vi "Measurement UI.vi"() -> ()   [LabVIEW 2021, in "Dialog Box UI.lvlib"]
uses:
  Dialog Box UI.lvlib
panel:
  in  "Clear":bool
  out "No?":bool
  out "Yes?":bool
  out "Ok?":bool
  in  "One Button DB":bool
  in  "Two Button DB":bool
  out "Selection":string
  in  "Three Button DB":bool
  out "Gender":string
  out "Location":u32(ring) items=["None", "Austin, TX", "New York City, NY", "Chicago, IL"]
  out "Name":string
  in  "Custom DB":bool
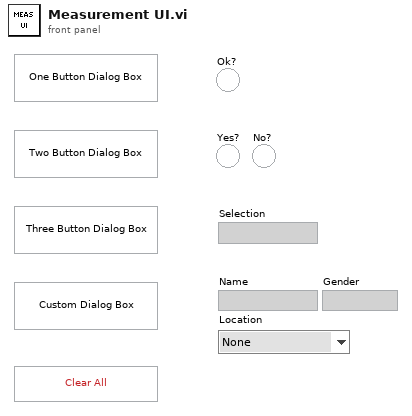
[diagram p1: front panel]
types:
  T1 = enum16{"Left Button", "Center Button", "Right Button", "Window Close"}
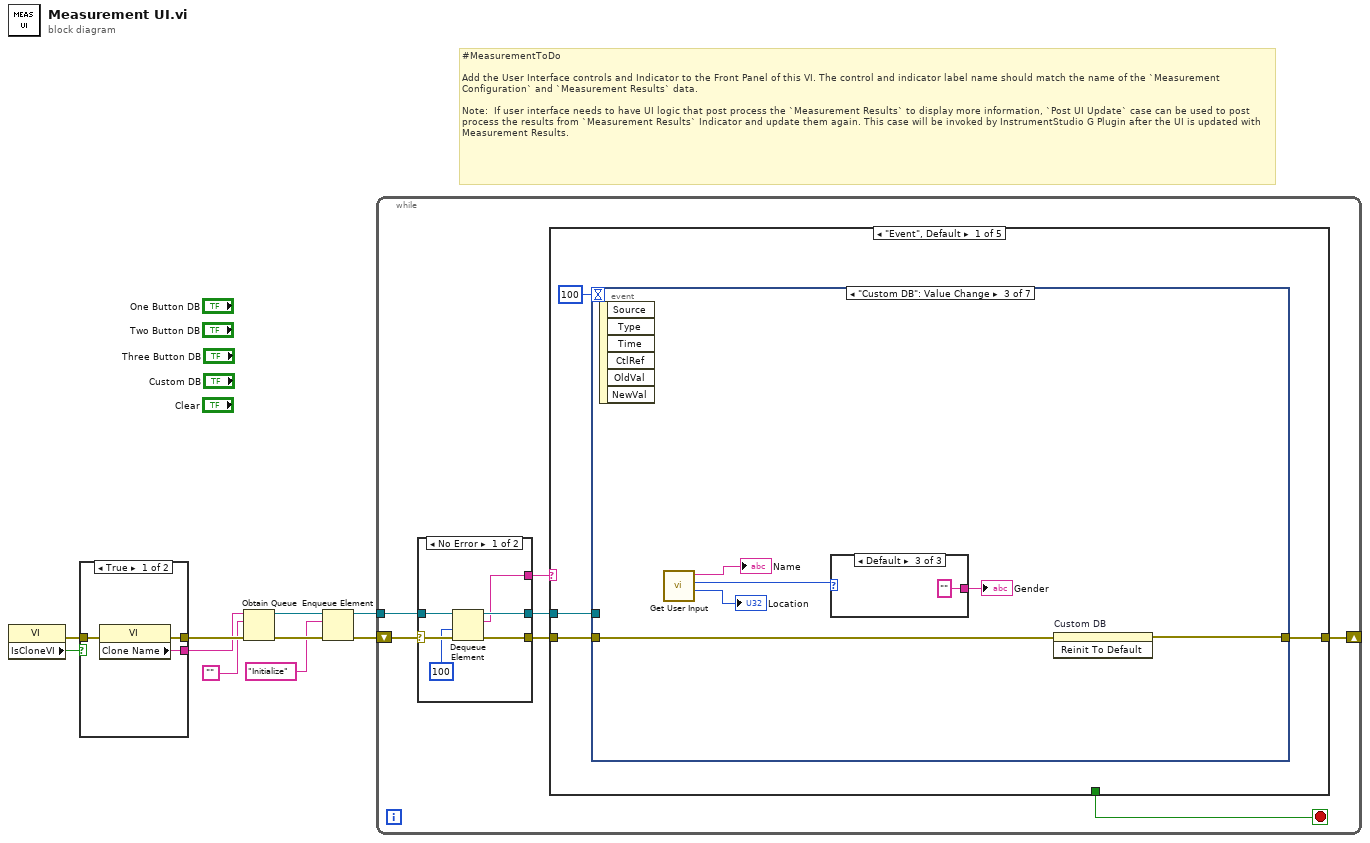
[diagram p0: block diagram]
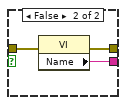
[diagram p2: hidden frame]
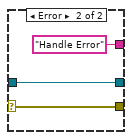
[diagram p3: hidden frame]
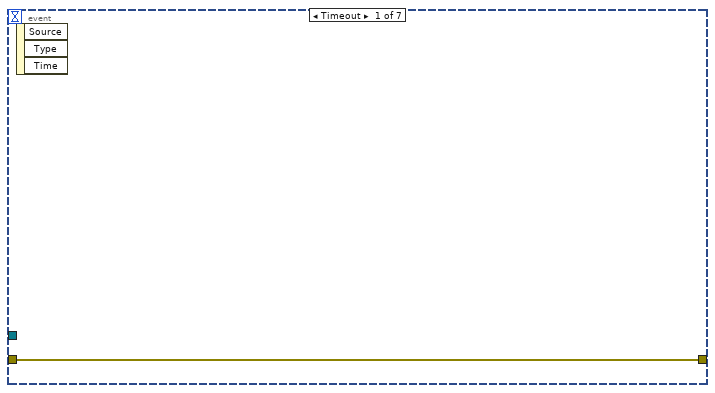
[diagram p4: hidden frame]
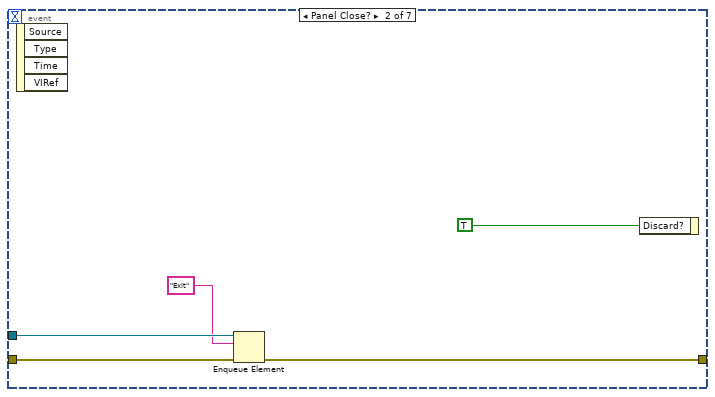
[diagram p5: hidden frame]
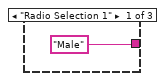
[diagram p6: hidden frame]
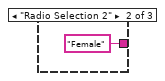
[diagram p7: hidden frame]
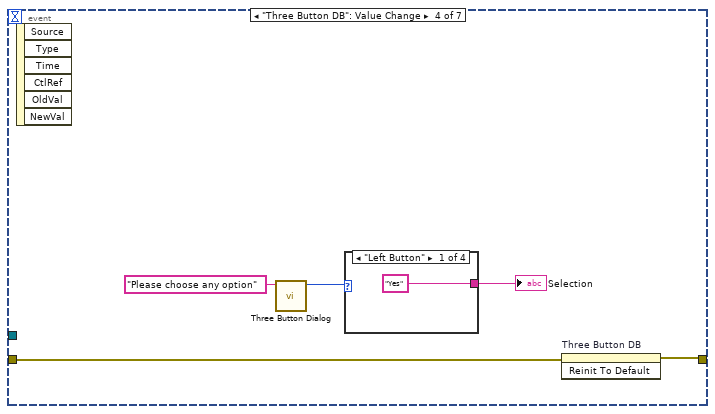
[diagram p8: hidden frame]
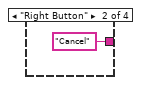
[diagram p9: hidden frame]
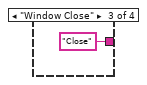
[diagram p10: hidden frame]
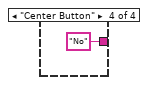
[diagram p11: hidden frame]
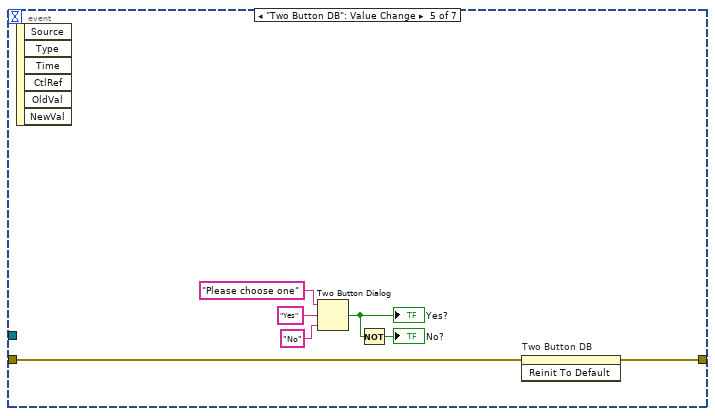
[diagram p12: hidden frame]
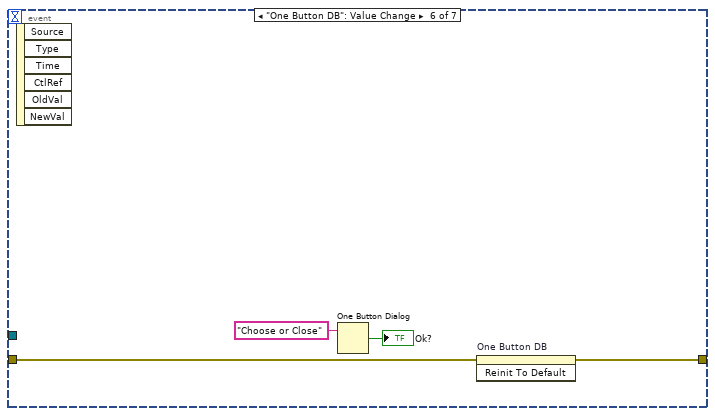
[diagram p13: hidden frame]
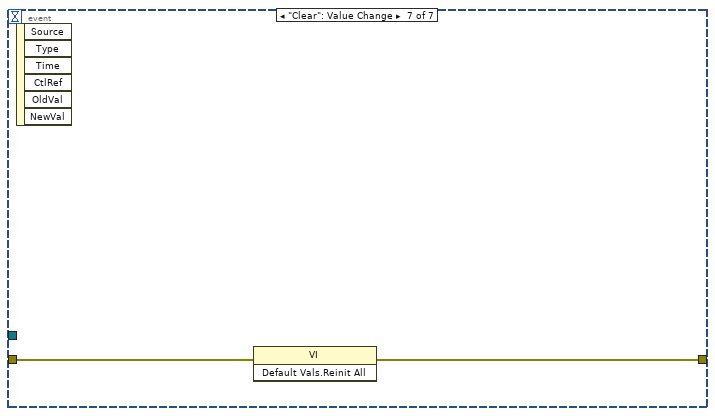
[diagram p14: hidden frame]
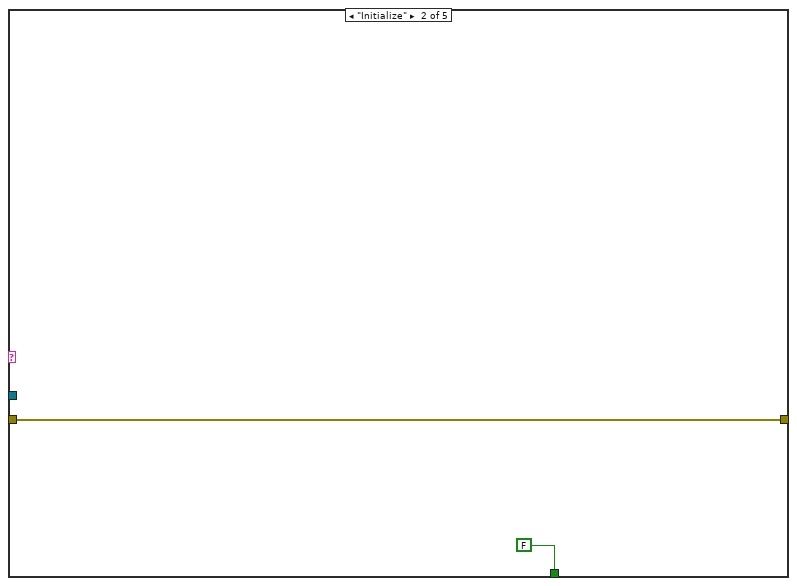
[diagram p15: hidden frame]
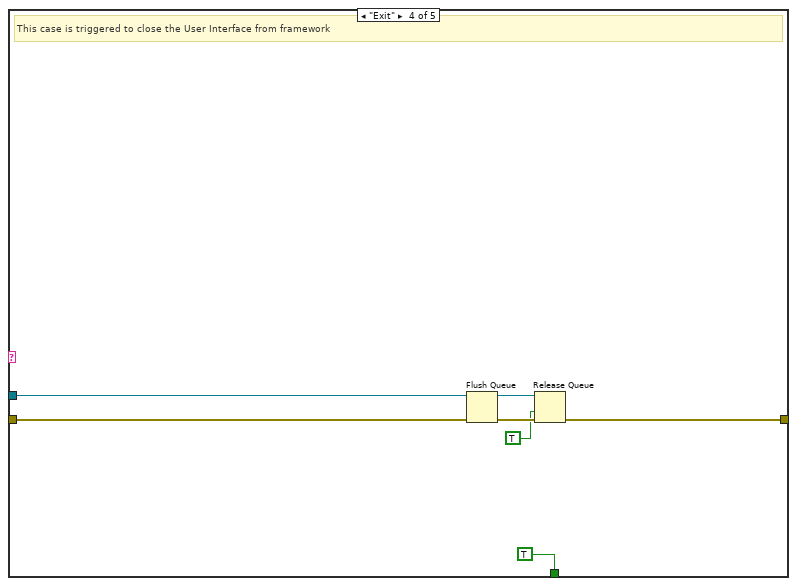
[diagram p17: hidden frame]
diagram:
  # "#MeasurementToDo  \n\nAdd the User Interface controls and Indicator to the Front Panel of this VI. The control and indicator label name should match the name of the `Measurement Configuration` and `Measurement Results` data.\n\nNote:  If user interface needs to have UI logic that post process the `Measurement Results` to display more information, `Post UI Update` case can be used to post process the results from `Measurement Results` Indicator and update them again. This case will be invoked by InstrumentStudio G Plugin after the UI is updated with Measurement Results."
  n1 = property class="VI"() -> (error out=w1:errorcluster, "IsCloneVI"=w2:bool)  [unwired: 2 in, 1 out]
  n2 = case shown="True" w2 {
    tunnel: [w13 w16] -> w10
    tunnel: [w12 w15] -> w9
    tunnel: w1 -> [w11 w14]
    frame True {
      n3 = property class="VI"(error in=w11) -> (error out=w13:errorcluster, "Clone Name"=w12:string)  [unwired: 1 in, 1 out]
    }
    frame False {
      n4 = property class="VI"(error in=w14) -> (error out=w16:errorcluster, "Name"=w15:string)  [unwired: 1 in, 1 out]
    }
  }
  n5 = Obtain Queue(name (unnamed)=w9, element data type="", error in (no error)=w10) -> (queue out=w6:refnum<queue>, error out=w8:errorcluster)  [unwired: 2 in, 1 out]
  n6 = Enqueue Element(queue=w6, element="Initialize", error in (no error)=w8) -> (queue out=w5:refnum<queue>, error out=w7:errorcluster)  [unwired: 1 in, 1 out]
  n7 = while {
    shift-right: [w18] -> _
    shift-left: w7 -> [w23]
    tunnel: w5 -> [w21]
    stop <- w17 stop-if-true
    n8 = case shown="No Error" w23 {
      selector: w23 -> [w29 w32]
      tunnel: [w28 w32] -> w22
      tunnel: w21 -> [w27 w31]
      tunnel: [w26 w31] -> w20
      tunnel: [w25 "Handle Error"] -> w19
      frame No Error {
        n9 = Dequeue Element(queue=w27, timeout in ms (-1)=100, error in (no error)=w29) -> (queue out=w26:refnum<queue>, element=w25:string, error out=w28:errorcluster)  [unwired: 1 out]
      }
      frame Error {
      }
    }
    n10 = case shown="\"Event\", Default" w19 {
      tunnel: w22 -> [w35 w75 w76 w83 w84]
      tunnel: w20 -> [w33 _ _ w81 _]
      tunnel: [w36 w75 w76 w78 w84] -> w18
      tunnel: [_ FALSE _ TRUE _] -> w17
      frame "Event", Default {
        n11 = event shown="[2] \"Custom DB\": Value Change" {
          selector: _ -> [_ _ _ _ _ _ _]
          dyn-events: _ -> [_ _ _ _ _ _ _]
          timeout: 100 -> [_ _ _ _ _ _ _]
          tunnel: [w37 w40 w47 w53 w65 w69 w72] -> w36
          tunnel: w35 -> [w37 w41 w48 w52 w66 w70 w73]
          tunnel: w33 -> [_ w39 _ _ _ _ _]
          event Timeout {
            n12 = event-data() -> ()  [unwired: 1 in, 3 out]
          }
          event Panel Close? {
            n13 = event-data() -> ()  [unwired: 1 in, 4 out]
            n14 = Enqueue Element(queue=w39, element="Exit", error in (no error)=w41) -> (error out=w40:errorcluster)  [unwired: 1 in, 2 out]
            n15 = event-data("Discard?"=TRUE) -> ()  [unwired: 1 in, 1 out]
          }
          event "Custom DB": Value Change {
            n16 = event-data() -> ()  [unwired: 1 in, 6 out]
            n17 = call "Get User Input.vi"() -> ("Location"=→"Location":u32, "Gender"=w44:enum32{"Radio Selection 1", "Radio Selection 2"}, "Name"=→"Name":string)  [unwired: 9 in]
            n18 = case shown="Default" w44 {
              tunnel: ["Male" ("Gender") "Female" ("Gender") "" ("Gender")] -> w43
              frame "Radio Selection 1" {
              }
              frame "Radio Selection 2" {
              }
              frame Default {
              }
            }
            "Gender" <- w43
            n19 = invoke on="Custom DB" class="Bool" method="Reinit To Default"(error in=w48) -> (error out=w47:errorcluster)  [unwired: 2 in, 2 out]
          }
          event "Three Button DB": Value Change {
            n20 = event-data() -> ()  [unwired: 1 in, 6 out]
            n21 = call <vilib>:"Three Button Dialog.vi"("message"="Please choose any option") -> ("Which Button?"=w55:T1)  [unwired: 10 in]
            n22 = case shown="\"Left Button\"" w55 {
              tunnel: ["Yes" ("Selection") "Cancel" ("Selection") "Close" ("Selection") "No" ("Selection")] -> w54
              frame "Left Button" {
              }
              frame "Right Button" {
              }
              frame "Window Close" {
              }
              frame "Center Button" {
              }
            }
            "Selection" <- w54
            n23 = invoke on="Three Button DB" class="Bool" method="Reinit To Default"(error in=w52) -> (error out=w53:errorcluster)  [unwired: 2 in, 2 out]
          }
          event "Two Button DB": Value Change {
            n24 = event-data() -> ()  [unwired: 1 in, 6 out]
            n25 = Two Button Dialog(message="Please choose one", 1:"No" ("F button name (\"Cancel\")"), 2:"Yes" ("T button name (\"OK\")")) -> (T button?=w62:bool)
            "Yes?" <- w62
            n26 = Not(x=w62) -> (.not. x?=→"No?":bool)
            n27 = invoke on="Two Button DB" class="Bool" method="Reinit To Default"(error in=w66) -> (error out=w65:errorcluster)  [unwired: 2 in, 2 out]
          }
          event "One Button DB": Value Change {
            n28 = event-data() -> ()  [unwired: 1 in, 6 out]
            n29 = One Button Dialog(message="Choose or Close") -> (true=→"Ok?":bool)  [unwired: 1 in]
            n30 = invoke on="One Button DB" class="Bool" method="Reinit To Default"(error in=w70) -> (error out=w69:errorcluster)  [unwired: 2 in, 2 out]
          }
          event "Clear": Value Change {
            n31 = event-data() -> ()  [unwired: 1 in, 6 out]
            n32 = invoke class="VI" method="Default Vals.Reinit All"(error in=w73) -> (error out=w72:errorcluster)  [unwired: 2 in, 2 out]
          }
        }
      }
      frame "Initialize" {
      }
      frame "Post UI Update" {
        # "This case will be triggered, after framework updates the User interface with result values."
      }
      frame "Exit" {
        # "This case is triggered to close the User Interface from framework"
        n33 = Flush Queue(queue=w81, error in (no error)=w83) -> (queue out=w80:refnum<queue>, error out=w79:errorcluster)  [unwired: 1 out]
        n34 = Release Queue(queue=w80, force destroy? (F)=TRUE, error in (no error)=w79) -> (error out=w78:errorcluster)  [unwired: 2 out]
      }
      frame "Handle Error" {
      }
    }
  }
